vi "setTics.vi"(7 "tics":T2, 9 "Axis":T1, 11 "String in":string) -> (0 "polarGrid":dbl, 2 "command":string, 3 "String out":string)   [LabVIEW 2012]
uses:
  tics.ctl
  axisName.ctl
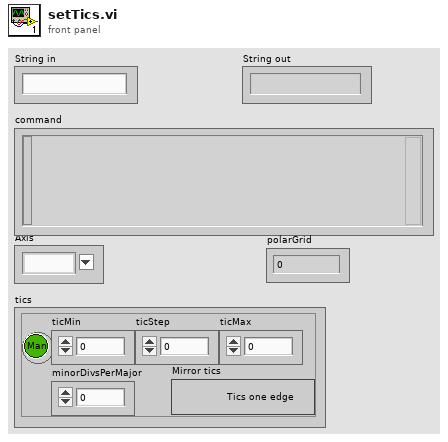
[diagram p1: front panel]
types:
  T1 = typedef "axisName.ctl" = string
  T2 = typedef "tics.ctl" = cluster{"Auto":bool, "ticMin":dbl, "ticStep":dbl, "ticMax":dbl, "minorDivsPerMajor":i32, "Mirror tics":bool}
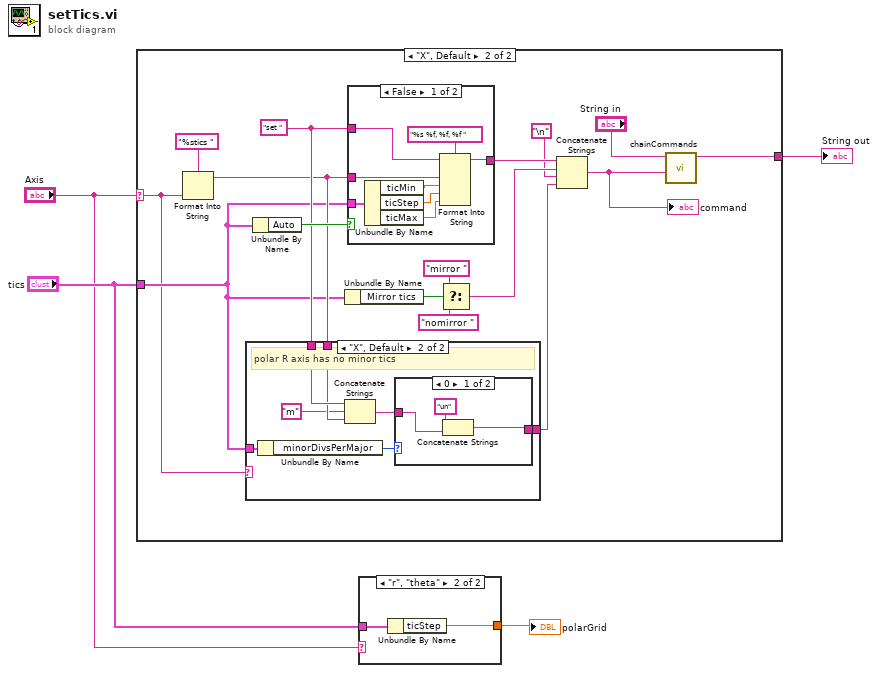
[diagram p0: block diagram]
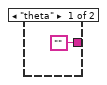
[diagram p2: hidden frame]
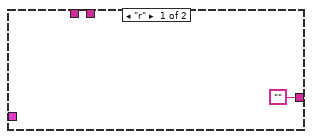
[diagram p3: hidden frame]
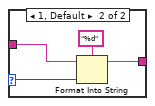
[diagram p4: hidden frame]
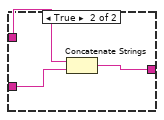
[diagram p5: hidden frame]
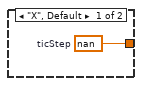
[diagram p6: hidden frame]
diagram:
  n1 = case shown="\"X\", Default" "Axis" {
    selector: "Axis" -> [_ w6]
    tunnel: ["" w14] -> w4
    tunnel: "tics" -> [_ w7]
    frame "theta" {
    }
    frame "X", Default {
      w11 = "set " ("format string")
      n2 = Format Into String(format string="%stics ", w6) -> (resulting string=w10:string)  [unwired: 2 in, 1 out]
      n3 = case shown="\"X\", Default" w6 {
        tunnel: w11 -> [_ w28]
        tunnel: w10 -> [_ w27]
        tunnel: ["" w24] -> w9
        tunnel: w7 -> [_ w23]
        frame "r" {
        }
        frame "X", Default {
          # "polar R axis has no minor tics"
          n4 = Unbundle By Name(w23) -> ("minorDivsPerMajor"=w29:i32)
          n5 = Concatenate Strings(w28, "m" ("string"), w27) -> (w25:string)
          n6 = case shown="0" w29 {
            selector: w29 -> [_ w34]
            tunnel: w25 -> [w32 w35]
            tunnel: [w31 w33] -> w24
            frame 0 {
              n7 = Concatenate Strings("un" ("string"), w32) -> (w31:string)
            }
            frame 1, Default {
              n8 = Format Into String(format string="%d", initial string=w35, w34) -> (resulting string=w33:string)  [unwired: 1 in, 1 out]
            }
          }
        }
      }
      n9 = Unbundle By Name(w7) -> ("Auto"=w15:bool)
      n10 = Unbundle By Name(w7) -> ("Mirror tics"=w17:bool)
      n11 = case shown="False" w15 {
        tunnel: [w44 w46] -> w20
        tunnel: w10 -> [w37 w47]
        tunnel: w7 -> [w42 _]
        tunnel: w11 -> [w38 w45]
        frame False {
          n12 = Unbundle By Name(w42) -> ("ticMin"=w39:dbl, "ticStep"=w41:dbl, "ticMax"=w40:dbl)
          n13 = Format Into String(format string="%s %f, %f, %f ", initial string=w38, w37, w39, w41, w40) -> (resulting string=w44:string)  [unwired: 1 in, 1 out]
        }
        frame True {
          n14 = Concatenate Strings(w45, w47) -> (w46:string)
        }
      }
      n15 = Select(t="mirror ", s=w17, f="nomirror ") -> (s? t:f=w21:string)
      n16 = Concatenate Strings(w20, w21, "\n", w9) -> (w12:string)
      "command" <- w12
      n17 = call "chainCommands.vi"("Command"=w12, "StringIn"="String in") -> ("StringOut"=w14:string)  [unwired: 9 in]
    }
  }
  "String out" <- w4
  n18 = case shown="\"r\", \"theta\"" "Axis" {
    tunnel: "tics" -> [_ w50]
    tunnel: [w48 w49] -> w2
    frame "X", Default {
      w48 = nan  # ticStep
    }
    frame "r", "theta" {
      n19 = Unbundle By Name(w50) -> ("ticStep"=w49:dbl)
    }
  }
  "polarGrid" <- w2
